vi "Ring Controls.vi"(6 "Cluster":T1={"Text Ring"=2, "Menu Ring"=21, "Text & Picture Ring"=11.0, "Picture Ring"=4} {"Text & Picture Ring" items=["Picture 1"=23.0, "Picture 2"=11.0, "Picture 3"=77.0, "Picture 4"=89.0]; "Menu Ring" items=["qqq"=120, "rrrrr"=52, "sssss"=21]; "Text Ring" items=["aaa", "bbb", "ccc", "ddd"]}, 8 "Picture Ring":u16(ring)=4, 9 "Text & Picture Ring":dbl(ring)=11.0 items=["Picture 1"=23.0, "Picture 2"=11.0, "Picture 3"=77.0, "Picture 4"=89.0], 10 "Menu Ring":u8(ring)=21 items=["qqq"=120, "rrrrr"=52, "sssss"=21], 11 "Text Ring":u32(ring)=2 items=["aaa", "bbb", "ccc", "ddd"]) -> ()   [LabVIEW 2009]
panel:
  in  "stop":bool
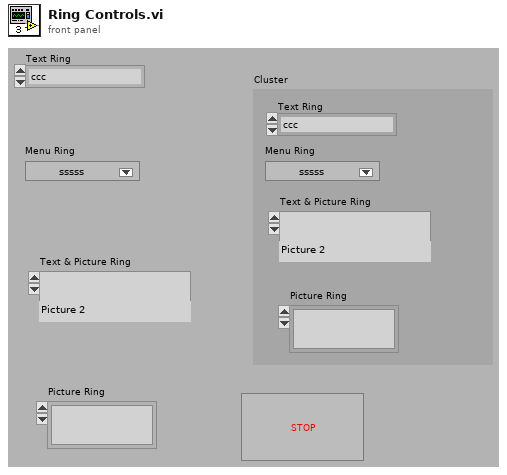
[diagram p1: front panel]
types:
  T1 = cluster{"Text Ring":u32, "Menu Ring":u8, "Text & Picture Ring":dbl, "Picture Ring":u16}
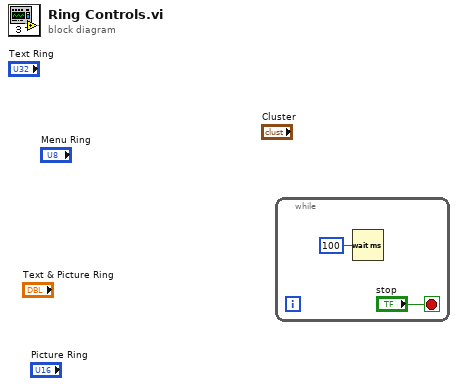
[diagram p0: block diagram]
diagram:
  n1 = while {
    stop <- "stop" stop-if-true
    n2 = Wait (ms)(milliseconds to wait=u32 100) -> ()  [unwired: 1 out]
  }
